vi "Visa name1.vi"() -> ()   [LabVIEW 2011]
panel:
  in  "VISA name":refnum<visa-resource-name>
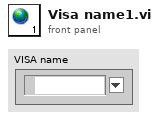
[diagram p1: front panel]
diagram:
